vi "ObtainAllMessageQues vxm.vi"(8 "error in":errorcluster, 9 "Error Que Name":string="Error", 10 "Motion Que Name":string="VXMService", 11 "Main Que Name":string="Main") -> (0 "error out":errorcluster, 3 "MessageQues":T1)   [LabVIEW 2018]
doc: "This VI creates and initializes all the message queues for your application. If your application requires more than one message queue, right-click the \"Message Queues\" constant above and select Open Type Def. Add the new Message Queue(s) to the type definition, then initialize them in this VI. \n\nThe que names are/can be used in the error handler loop. It can use the names to provide unique error handling for selected state machine loops.\n\nBolder Software LLC"
uses:
  MultipleMessageQues vxm.ctl
  MessageQue.ctl
  MessageCluster.ctl
  MessageQue.lvlib
panel:
  in  "DAQ Que Name":string="DAQ"
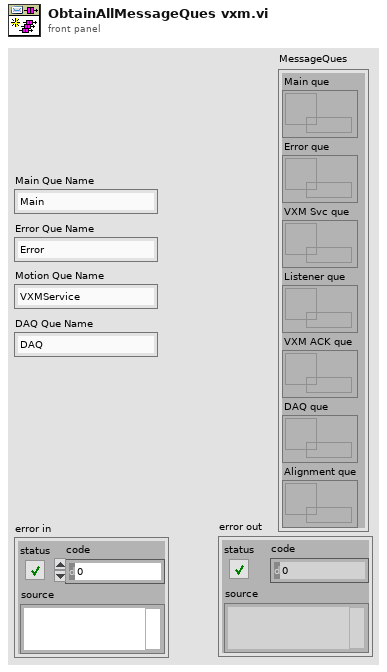
[diagram p1: front panel]
types:
  T1 = typedef "MultipleMessageQues vxm.ctl" = cluster{"Main que":T2, "Error que":T2, "VXM Svc que":T2, "Listener que":T2, "VXM ACK que":T2, "DAQ que":T2, "Alignment que":T2}
  T2 = typedef "MessageQue.lvlib/MessageQue.ctl" = refnum<queue>
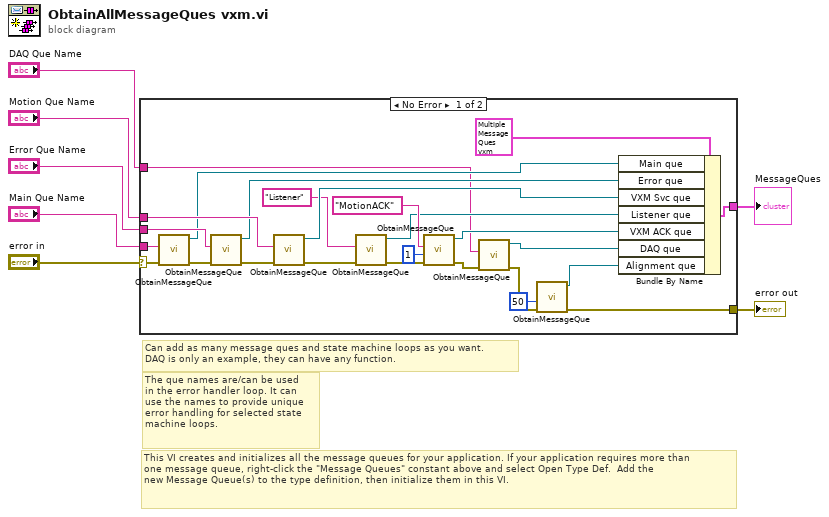
[diagram p0: block diagram]
diagram:
  # "The que names are/can be used\nin the error handler loop. It can\nuse the names to provide unique\nerror handling for selected state\nmachine loops."
  # "Can add as many message ques and state machine loops as you want. \nDAQ is only an example, they can have any function."
  # "This VI creates and initializes all the message queues for your application. If your application requires more than \none message queue, right-click the \"Message Queues\" constant above and select Open Type Def.  Add the \nnew Message Queue(s) to the type definition, then initialize them in this VI."
  n1 = case shown="No Error" "error in" {
    selector: "error in" -> [w26 w33]
    tunnel: "Main Que Name" -> [w32 _]
    tunnel: [w31 _] -> w4
    tunnel: "Error Que Name" -> [w30 _]
    tunnel: "Motion Que Name" -> [w29 _]
    tunnel: [w9 w33] -> w6
    tunnel: "DAQ Que Name" -> [w15 _]
    frame No Error {
      n2 = call "ObtainMessageQue.vi"("error in"=w26, "Name"=w32) -> ("error out"=w27:errorcluster, "message que out"=w24:T2)  [unwired: 6 in, 2 out]
      n3 = call "ObtainMessageQue.vi"("error in"=w27, "Name"=w30) -> ("error out"=w28:errorcluster, "message que out"=w23:T2)  [unwired: 6 in, 2 out]
      n4 = call "ObtainMessageQue.vi"("error in"=w28, "Name"=w29) -> ("error out"=w19:errorcluster, "message que out"=w22:T2)  [unwired: 6 in, 2 out]
      n5 = call "ObtainMessageQue.vi"("error in"=w19, "Name"="Listener") -> ("error out"=w18:errorcluster, "message que out"=w17:T2)  [unwired: 6 in, 2 out]
      n6 = call "ObtainMessageQue.vi"("error in"=w18, "max queue size (-1, unlimited)"=1, "Name"="MotionACK") -> ("error out"=w13:errorcluster, "message que out"=w16:T2)  [unwired: 5 in, 2 out]
      n7 = call "ObtainMessageQue.vi"("error in"=w13, "Name"=w15) -> ("error out"=w10:errorcluster, "message que out"=w14:T2)  [unwired: 6 in, 2 out]
      n8 = call "ObtainMessageQue.vi"("error in"=w10, "max queue size (-1, unlimited)"=50) -> ("error out"=w9:errorcluster, "message que out"=w11:T2)  [unwired: 6 in, 2 out]
      n9 = Bundle By Name(cluster=T1 {"Main que"=refnum, "Error que"=refnum, "VXM Svc que"=refnum, "Listener que"=refnum, "VXM ACK que"=refnum, "DAQ que"=refnum, "Alignment que"=refnum} ("MessageQues"), "Main que"=w24, "Error que"=w23, "VXM Svc que"=w22, "Listener que"=w17, "VXM ACK que"=w16, "DAQ que"=w14, "Alignment que"=w11) -> (w31:T1)
    }
    frame Error {
    }
  }
  "error out" <- w6
  "MessageQues" <- w4
